vi "Create Folder if Non Existent.vi"(8 "error in (no error)":errorcluster, 11 "Folder to Create":path) -> (0 "error out":errorcluster, 3 "New Path Out":path)   [LabVIEW 2015]
doc: "Create a new folder if one does not already exist."
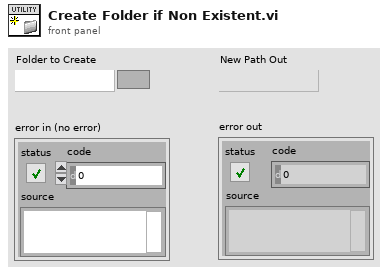
[diagram p1: front panel]
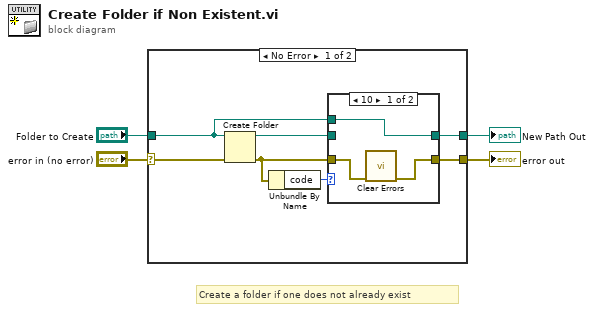
[diagram p0: block diagram]
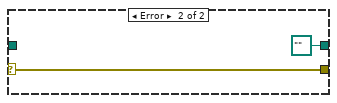
[diagram p3: hidden frame]
diagram:
  # "Create a folder if one does not already exist"
  n1 = case shown="No Error" "error in (no error)" {
    selector: "error in (no error)" -> [w11 w18]
    tunnel: "Folder to Create" -> [w5 _]
    tunnel: [w7 path "" ("created path")] -> w2
    tunnel: [w6 w18] -> w1
    frame No Error {
      n2 = Create Folder(path (use dialog)=w5, error in=w11) -> (created path=w8:path, error out=w10:errorcluster)  [unwired: 1 in, 1 out]
      n3 = Unbundle By Name(w10) -> ("code"=w9:i32)
      n4 = case shown="10" w9 {
        tunnel: w10 -> [w14 w16]
        tunnel: [w13 w16] -> w6
        tunnel: w8 -> [_ w15]
        tunnel: [w12 w15] -> w7
        tunnel: w5 -> [w12 _]
        frame 10 {
          n5 = call <vilib>:"Clear Errors.vi"("error in (no error)"=w14) -> ("error out"=w13:errorcluster)  [unwired: 5 in, 1 out]
        }
        frame Default {
        }
      }
    }
    frame Error {
    }
  }
  "error out" <- w1
  "New Path Out" <- w2
